vi "HindbrainMain.vi"(7 "Notifiers":T1, 8 "XBEE Refference":refnum<visa-resource-name>) -> (3 "String Received":string)   [LabVIEW 2013]
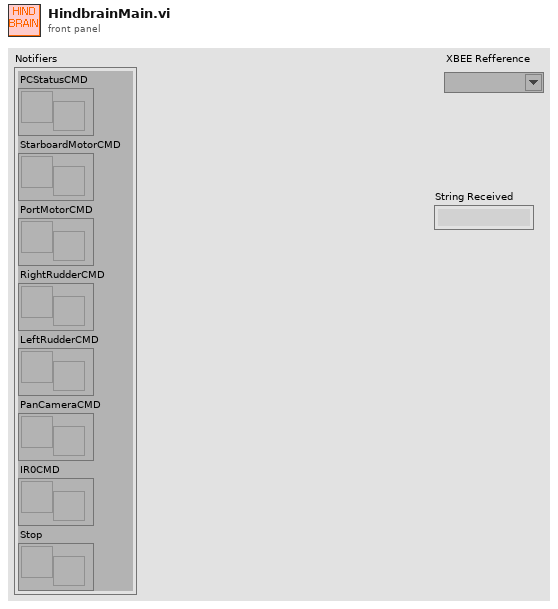
[diagram p1: front panel]
types:
  T1 = cluster{"PCStatusCMD":refnum<notifier>, "StarboardMotorCMD":refnum<notifier>, "PortMotorCMD":refnum<notifier>, "RightRudderCMD":refnum<notifier>, "LeftRudderCMD":refnum<notifier>, "PanCameraCMD":refnum<notifier>, "IR0CMD":refnum<notifier>, "Stop":refnum<notifier>}
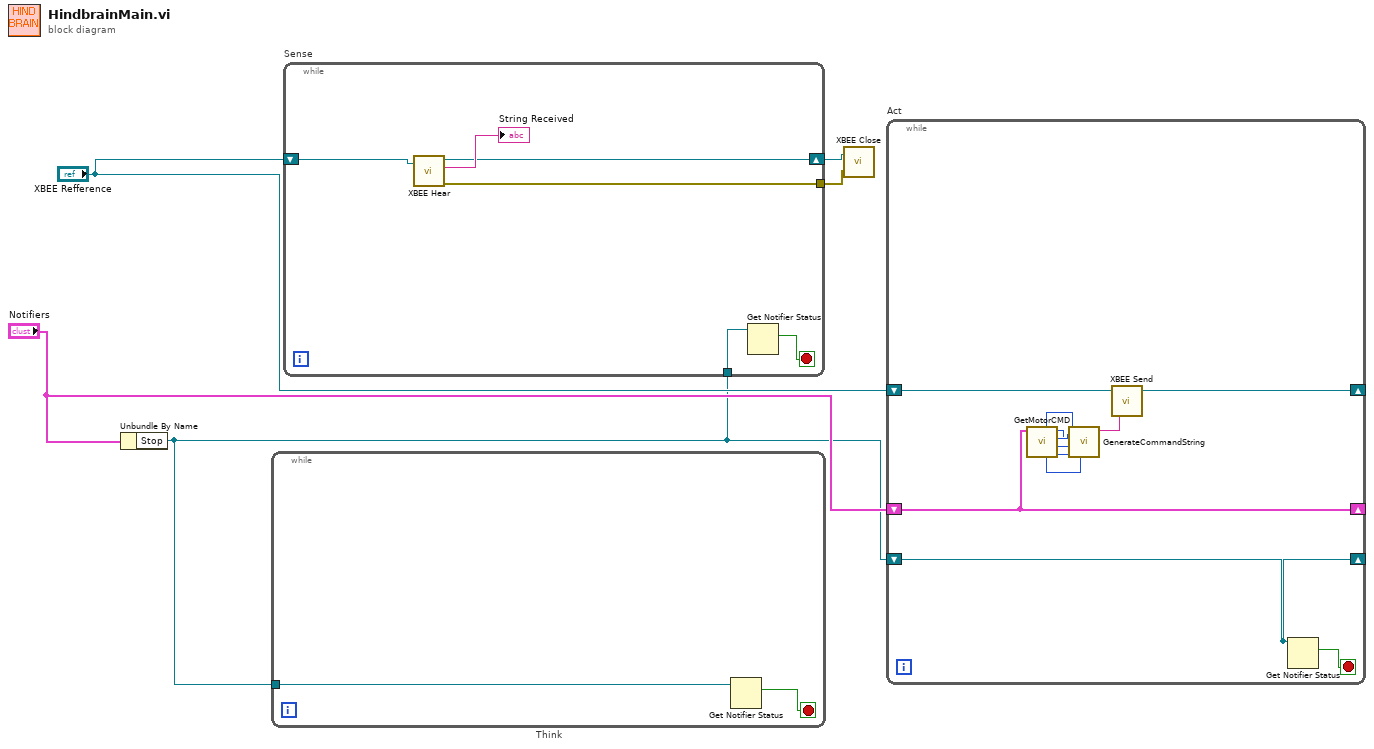
[diagram p0: block diagram]
diagram:
  n1 = Unbundle By Name("Notifiers") -> ("Stop"=w3:refnum<notifier>)
  n2 = while "Think" {
    tunnel: w3 -> [w6]
    stop <- w7 stop-if-true
    n3 = Get Notifier Status(notifier=w6) -> (current notification=w7:bool)  [unwired: 1 in, 4 out]
  }
  n4 = while "Sense" {
    tunnel: w3 -> [w11]
    tunnel: [w8] -> w1
    shift-right: [w9] -> w2
    shift-left: "XBEE Refference" -> [w13]
    stop <- w12 stop-if-true
    n5 = call "XBEE Hear.vi"("VISA resource name"=w13) -> ("VISA resource name out"=w9:refnum<visa-resource-name>, "String Received"=→"String Received":string, "error out"=w8:errorcluster)  [unwired: 1 in, 1 out]
    n6 = Get Notifier Status(notifier=w11) -> (current notification=w12:bool)  [unwired: 1 in, 4 out]
  }
  n7 = call "XBEE Close.vi"("error in (no error)"=w1, "VISA resource name"=w2) -> ()
  n8 = while "Act" {
    shift-right: [w16] -> _
    shift-left: "Notifiers" -> [w16]
    shift-right: [w15] -> _
    shift-left: "XBEE Refference" -> [w25]
    shift-right: [w14] -> _
    shift-left: w3 -> [w14]
    stop <- w17 stop-if-true
    n9 = call "GetMotorCMD.vi"("Notifiers"=w16) -> ("PanCameraCMD"=w24:i32, "LeftRudderCMD"=w23:i32, "StarboardMotorCMD"=w22:i32, "PCStatusCMD"=w21:i32, "RightRudderCMD"=w19:i32, "PortMotorCMD"=w20:i32)  [unwired: 5 in]
    n10 = call "GenerateCommandString.vi"("Right Rubber"=w19, "Port\nMotor"=w22, "Pan Camera"=w24, "Left Rudder"=w23, "Starboard\nMotor"=w21, "PC Status"=w20) -> ("CommandString"=w18:string)  [unwired: 5 in]
    n11 = call "XBEE Send.vi"("String"=w18, "VISA resource name"=w25) -> ("VISA resource name out"=w15:refnum<visa-resource-name>)  [unwired: 1 in, 2 out]
    n12 = Get Notifier Status(notifier=w14) -> (current notification=w17:bool)  [unwired: 1 in, 4 out]
  }
